vi "update_params.vi"(1 "Polarization":dbl, 2 "Input cluster":T1, 3 "Field":dbl, 4 "Dose":dbl, 5 "Frequency":dbl, 6 "Time":i64) -> (0 "Output cluster":T1)   [LabVIEW 2015]
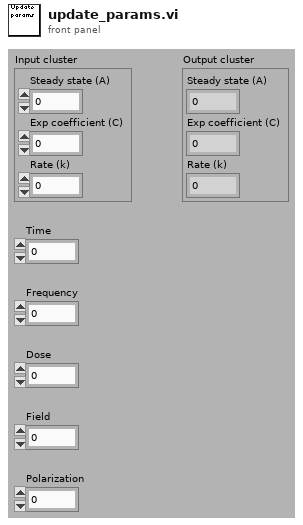
[diagram p1: front panel]
types:
  T1 = cluster{"Steady state (A)":dbl, "Exp coefficient (C)":dbl, "Rate (k)":dbl}
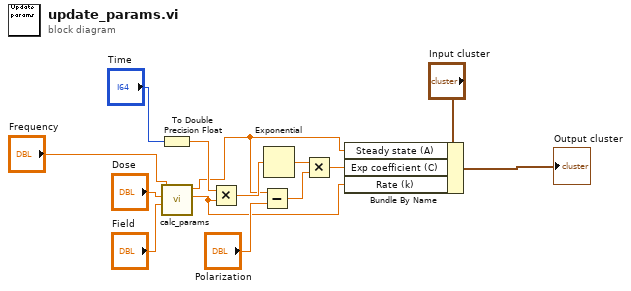
[diagram p0: block diagram]
diagram:
  n1 = To Double Precision Float(number="Time") -> (double precision float=w9:dbl)
  n2 = call "calc_params.vi"("Field"="Field", "Dose"="Dose", "Frequency"="Frequency") -> ("K value (rate)"=w5:dbl, "Steady state"=w1:dbl)  [unwired: 1 in, 2 out]
  n3 = Multiply(x=w9, y=w5) -> (x*y=w7:dbl)
  n4 = Subtract(x=w1, y="Polarization") -> (x-y=w12:dbl)
  n5 = Exponential(1:w7) -> (0:w10:dbl)
  n6 = Multiply(x=w10, y=w12) -> (x*y=w13:dbl)
  n7 = Bundle By Name(cluster="Input cluster", "Steady state (A)"=w1, "Exp coefficient (C)"=w13, "Rate (k)"=w5) -> (→"Output cluster":T1)
